vi "get array data.vi"(8 "error in (no error)":errorcluster, 11 "JSON Value in":refnum<class "JSON Value.lvclass">) -> (0 "error out":errorcluster, 3 "JSON Array out":refnum<class "JSON Value.lvclass">[](array[class]))   [LabVIEW 2016, in "JSON Value.lvclass"]
uses:
  JSON Value.lvclass
  JSON Value.lvclass/JSON Value.ctl
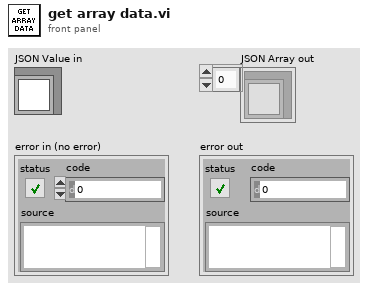
[diagram p1: front panel]
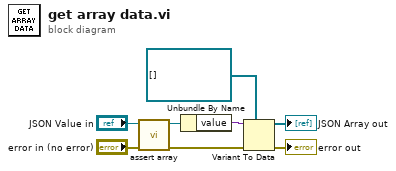
[diagram p0: block diagram]
diagram:
  n1 = call "assert array.vi"("error in (no error)"="error in (no error)", "JSON Value in"="JSON Value in") -> ("error out"=w3:errorcluster, "JSON Value out"=w1:refnum<class "JSON Value.lvclass">)  [unwired: 8 in]
  n2 = Unbundle By Name(w1) -> ("value"=w4:variant)
  n3 = Variant To Data(error in=w3, type=refnum<class "JSON Value.lvclass">[] [] ("JSON Array in"), Variant=w4) -> (data=→"JSON Array out":refnum<class "JSON Value.lvclass">[], error out=→"error out":errorcluster)
